vi "PlateReaderTimeTest.vi"() -> ()   [LabVIEW 2014]
uses:
  EventHandleInstrumentStatusChangedData.ctl
  EventHandleErrorReportData.ctl
  EventHandleCommandCompletedData.ctl
  C:/Program Files (x86)/Molecular Devices/SoftMax Pro 6.5.1 Automation SDK/SoftMaxPro.AutomationClient.dll
  Program Files (x86)/Molecular Devices/SoftMax Pro 6.5.1 Automation SDK/SoftMaxPro.AutomationClient.dll
  PlateReaderGlobal.vi
panel:
  out "Destruct Error":errorcluster
  out "String":string
  in  "ColumnName":string="1"
  out "Offsets":dbl[](array[numeric])
  in  "READ STOP":bool
  in  "READ START":bool
  in  "stop":bool
  out "Status":string
  out "ErrorReportQueue":T1[](array[typedef])
  out "CommandCompleteQueue":T2[](array[typedef])
  out "GetDataCopy":i32
  out "CommandCompleted":T2
  out "ErrorReport":T1
  out "InstrumentStatusChanged":T3
  out "StartRead":i32
  out "Initialize":bool
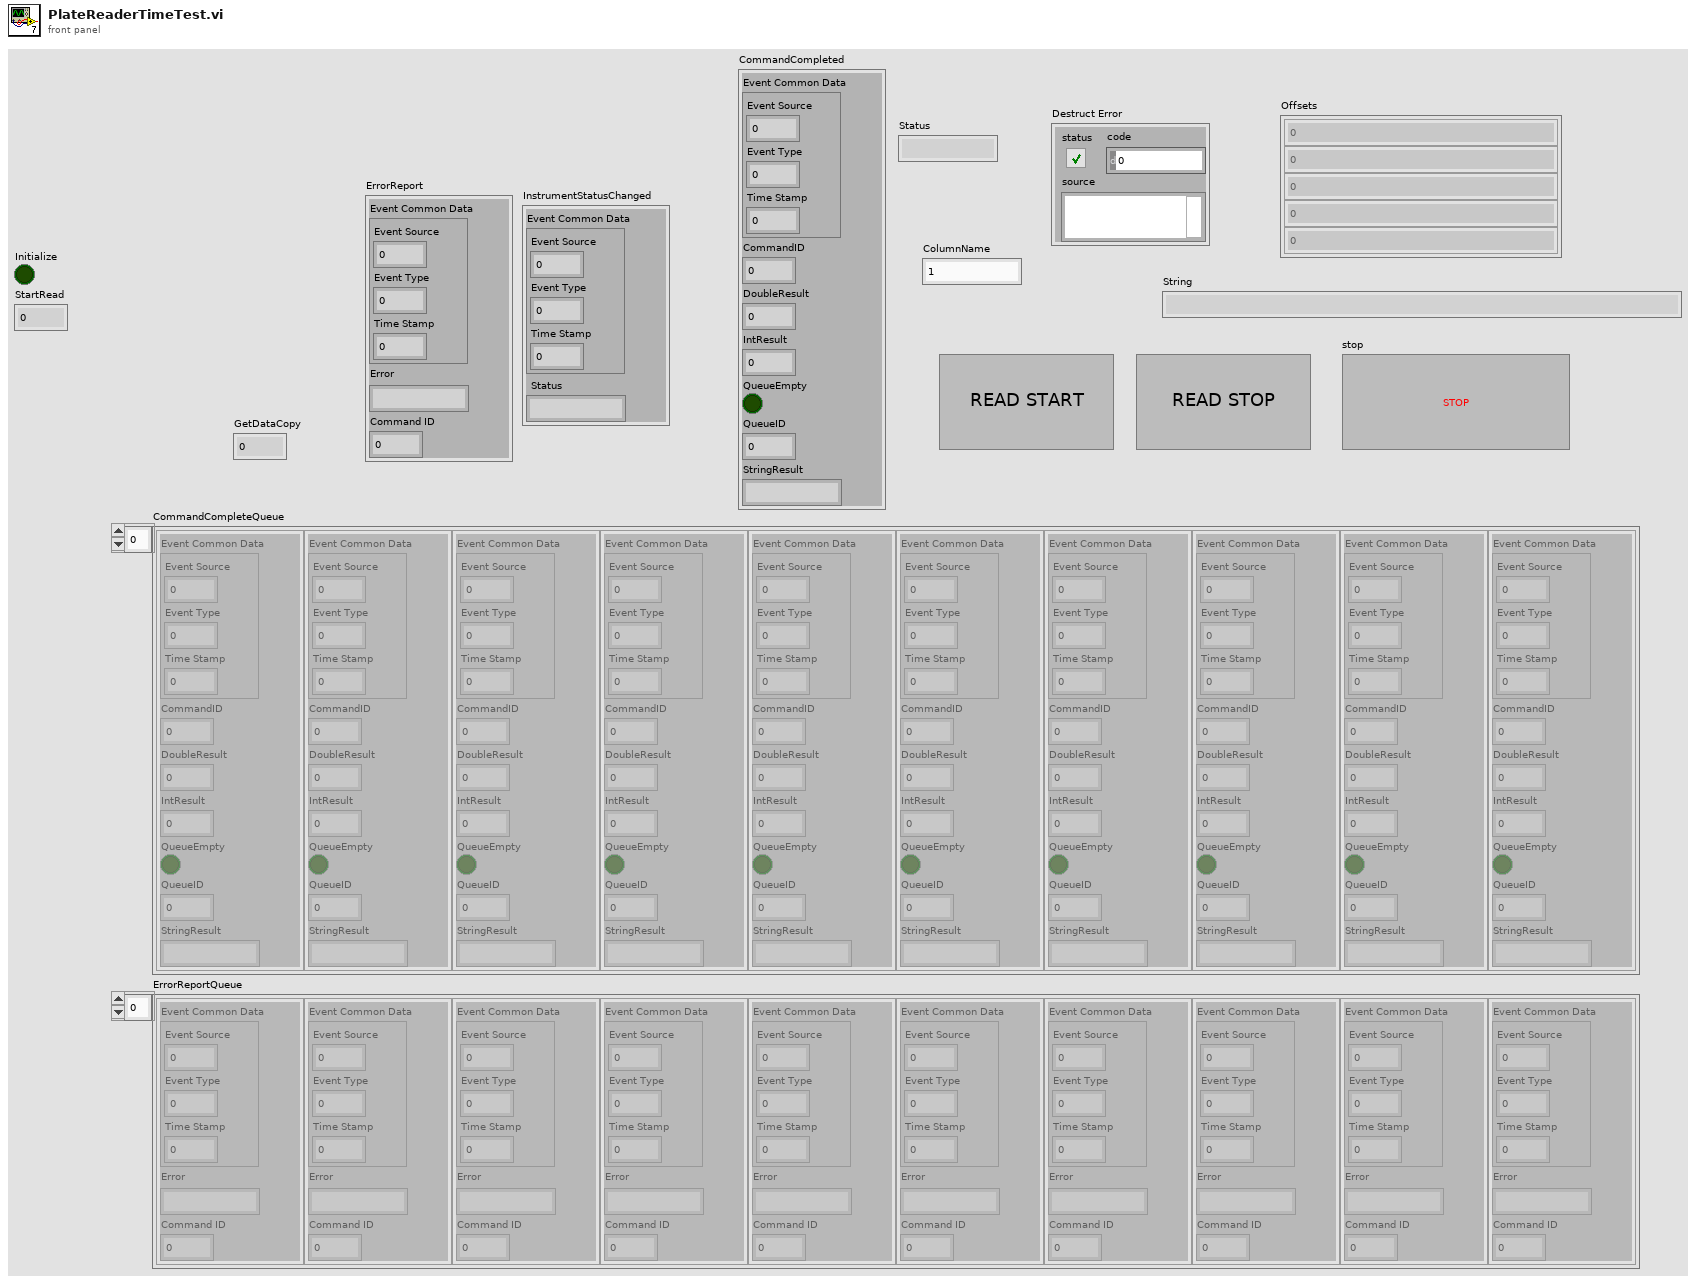
[diagram p1: front panel]
types:
  T1 = typedef "EventHandleErrorReportData.ctl" = cluster{"Event Common Data":cluster{"Event Source":i32, "Event Type":u32, "Time Stamp":u32}, "Error":string, "Command ID":i32}
  T2 = typedef "EventHandleCommandCompletedData.ctl" = cluster{"Event Common Data":cluster{"Event Source":i32, "Event Type":u32, "Time Stamp":u32}, "CommandID":i32, "DoubleResult":dbl, "IntResult":i32, "QueueEmpty":bool, "QueueID":i32, "StringResult":string}
  T3 = typedef "EventHandleInstrumentStatusChangedData.ctl" = cluster{"Event Common Data":cluster{"Event Source":i32, "Event Type":u32, "Time Stamp":u32}, "Status":string}
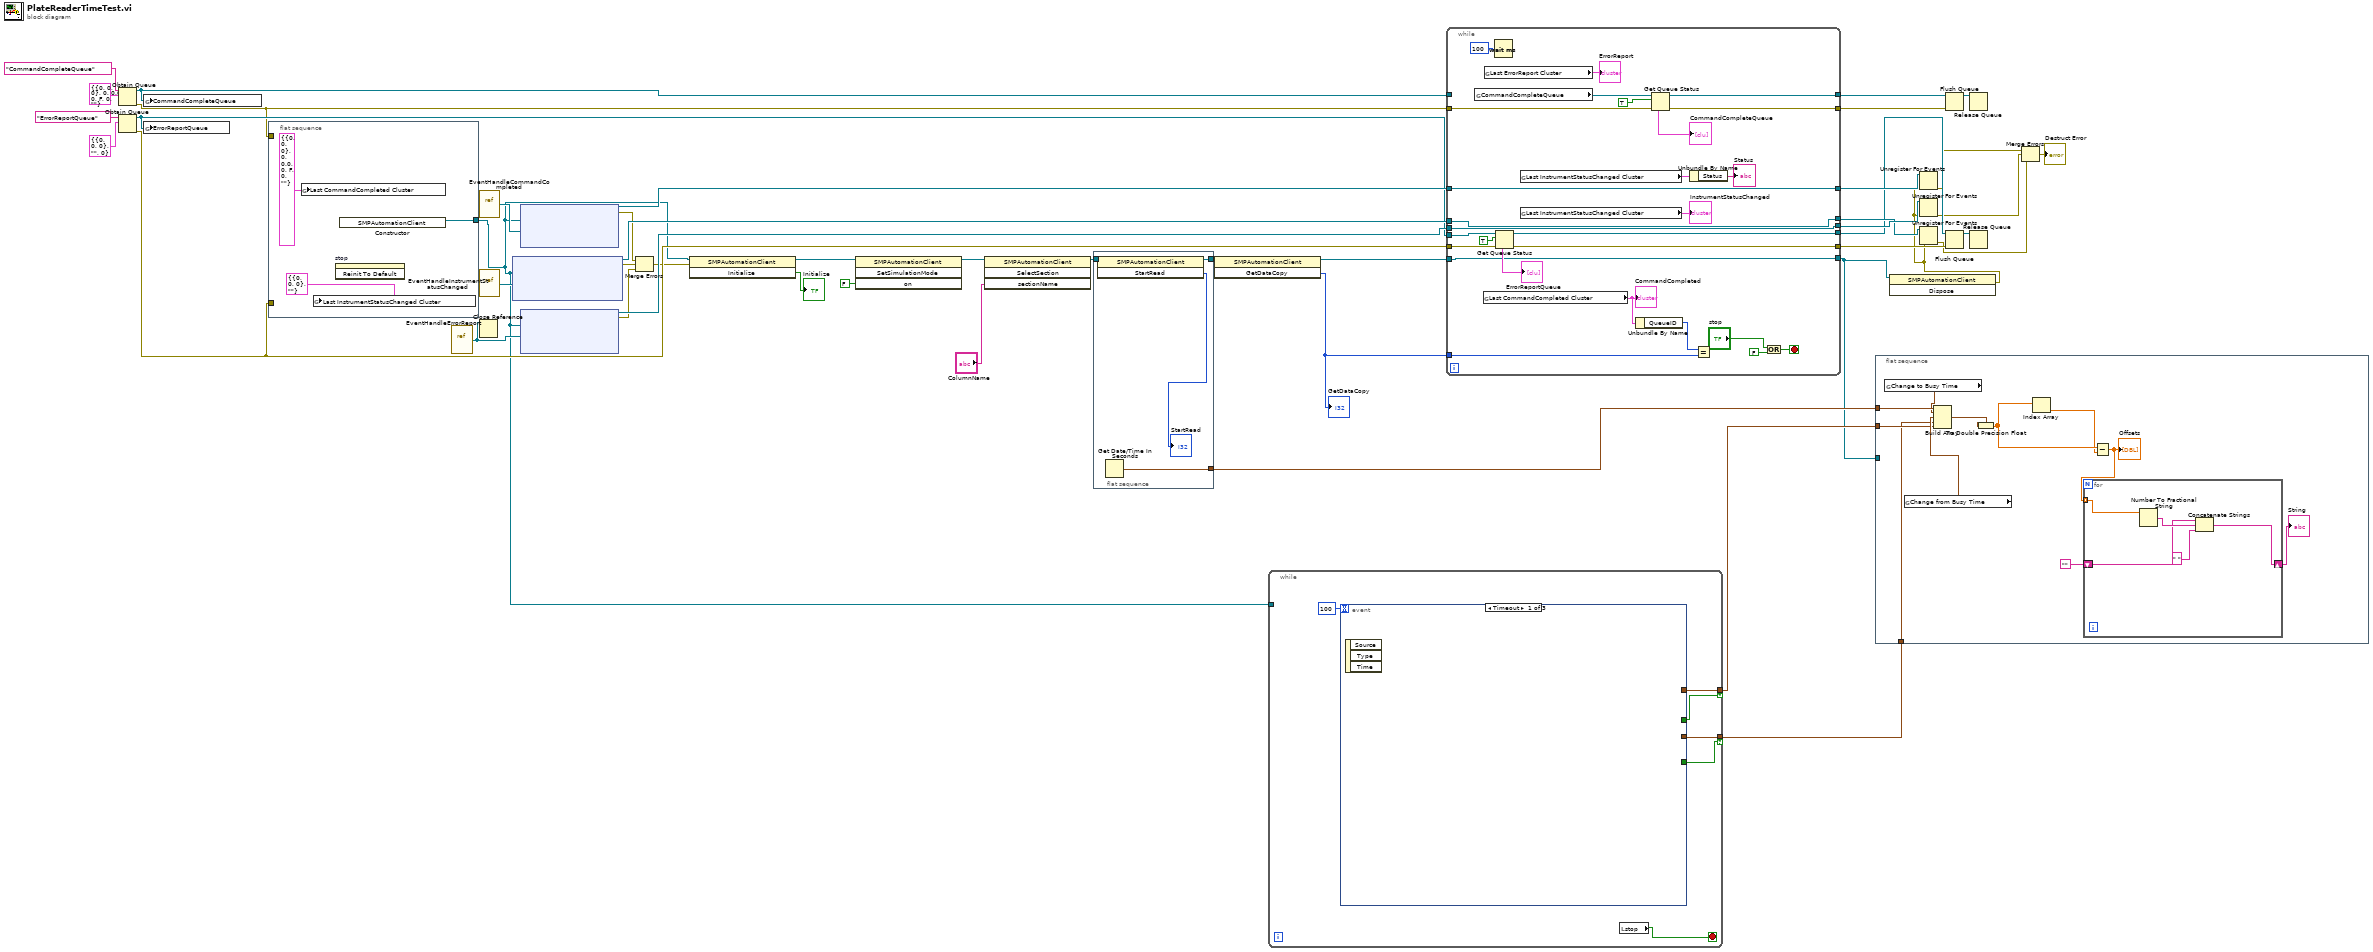
[diagram p0: block diagram]
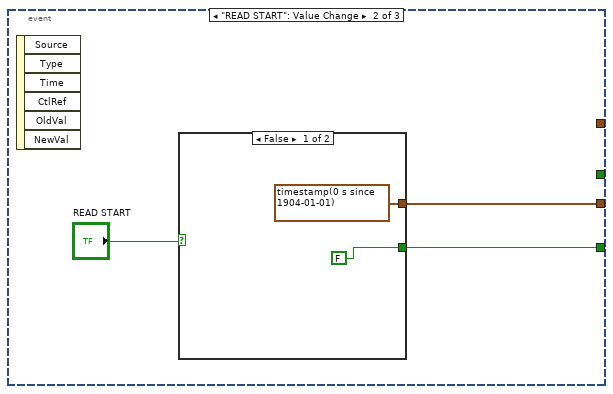
[diagram p2: hidden frame]
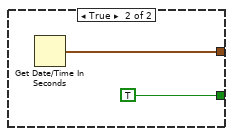
[diagram p3: hidden frame]
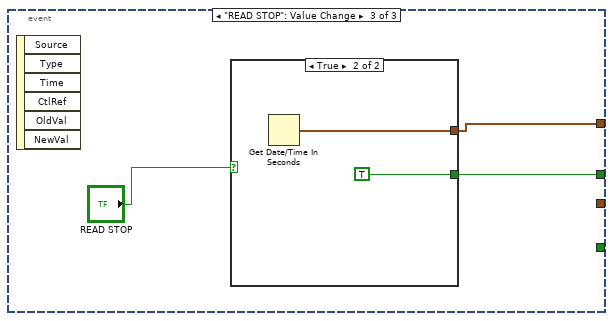
[diagram p4: hidden frame]
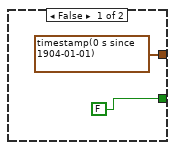
[diagram p5: hidden frame]
diagram:
  n1 = Obtain Queue(name (unnamed)="CommandCompleteQueue", element data type=T2 {"Event Common Data"={"Event Source"=0, "Event Type"=0, "Time Stamp"=0}, "CommandID"=0, "DoubleResult"=0.0, "IntResult"=0, "QueueEmpty"=FALSE, "QueueID"=0, "StringResult"=""} ("Event Data Cluster")) -> (queue out=w26:refnum<queue>, error out=w21:errorcluster)  [unwired: 3 in, 1 out]
  n2 = Obtain Queue(name (unnamed)="ErrorReportQueue", element data type=T1 {"Event Common Data"={"Event Source"=0, "Event Type"=0, "Time Stamp"=0}, "Error"="", "Command ID"=0} ("ErrorReport Data")) -> (queue out=w24:refnum<queue>, error out=w22:errorcluster)  [unwired: 3 in, 1 out]
  n3 = global write "PlateReaderGlobal.vi" "CommandCompleteQueue"(w26) -> ()
  n4 = global write "PlateReaderGlobal.vi" "ErrorReportQueue"(w24) -> ()
  n5 = flat-sequence {
    tunnel: [w49] -> w8
    tunnel: w22 -> [_]
    tunnel: w21 -> [_]
    frame #0 {
      n6 = global write "PlateReaderGlobal.vi" "Last CommandCompleted Cluster"(T2 {"Event Common Data"={"Event Source"=0, "Event Type"=0, "Time Stamp"=0}, "CommandID"=0, "DoubleResult"=0.0, "IntResult"=0, "QueueEmpty"=FALSE, "QueueID"=0, "StringResult"=""} ("Last CommandCompleted Cluster")) -> ()
      n7 = global write "PlateReaderGlobal.vi" "Last InstrumentStatusChanged Cluster"(T3 {"Event Common Data"={"Event Source"=0, "Event Type"=0, "Time Stamp"=0}, "Status"=""} ("Last InstrumentStatusChanged Cluster")) -> ()
      n8 = invoke on="stop" class="Bool (strict)" method="Reinit To Default"() -> ()  [unwired: 3 in, 3 out]
      n9 = constructor class="SMPAutomationClient"() -> (reference out=w49:refnum<k24>)  [unwired: 3 in, 2 out]
    }
  }
  n10 = vi-ref "EventHandleErrorReport.vi"() -> ("vi reference"=w35:refnum<vi>)
  n11 = vi-ref "EventHandleCommandCompleted.vi"() -> ("vi reference"=w40:refnum<vi>)
  n12 = vi-ref "EventHandleInstrumentStatusChanged.vi"() -> ("vi reference"=w39:refnum<vi>)
  n13 = Close Reference(reference=w35) -> ()  [unwired: 1 in, 1 out]
  n14 = node(w8, w39) -> (w41:refnum<k27>, w37:errorcluster)  [unwired: 3 in]
  n15 = node(w8, w40) -> (w45:refnum<k27>, w38:errorcluster)  [unwired: 3 in]
  n16 = node(w8, w35) -> (w43:refnum<k27>, w36:errorcluster)  [unwired: 3 in]
  n17 = Merge Errors(w38, w37, w36) -> (w20:errorcluster)
  n18 = invoke class="SMPAutomationClient" method="Initialize"(reference=w8, error in=w20) -> (reference out=w13:refnum<k24>, "Initialize"=→"Initialize":bool)  [unwired: 1 in, 1 out]
  n19 = invoke class="SMPAutomationClient" method="SetSimulationMode"(reference=w13, "on"=FALSE) -> (reference out=w17:refnum<k24>)  [unwired: 2 in, 3 out]
  n20 = invoke class="SMPAutomationClient" method="SelectSection"(reference=w17, "sectionName"="ColumnName") -> (reference out=w16:refnum<k24>)  [unwired: 2 in, 3 out]
  n21 = flat-sequence {
    tunnel: w16 -> [w53]
    tunnel: [w52] -> w15
    tunnel: [w50] -> w12
    frame #0 {
      n22 = invoke class="SMPAutomationClient" method="StartRead"(reference=w53) -> (reference out=w52:refnum<k24>, "StartRead"=→"StartRead":i32)  [unwired: 2 in, 1 out]
      n23 = Get Date/Time In Seconds() -> (seconds since 1Jan1904=w50:timestamp)
    }
  }
  n24 = invoke class="SMPAutomationClient" method="GetDataCopy"(reference=w15) -> (reference out=w7:refnum<k24>, "GetDataCopy"=w14:i32)  [unwired: 2 in, 1 out]
  "GetDataCopy" <- w14
  n25 = while {
    tunnel: [w60] -> w10 if=w59
    tunnel: [w58] -> w11 if=w57
    tunnel: [w54] -> _
    tunnel: w8 -> [w54]
    stop <- w56 stop-if-true
    n26 = event shown="[0] Timeout" {
      selector: _ -> [_ _ _]
      dyn-events: _ -> [_ _ _]
      timeout: 100 -> [_ _ _]
      tunnel: [_ w62 _] -> w60
      tunnel: [_ w61 _] -> w59
      tunnel: [_ _ w69] -> w58
      tunnel: [_ _ w68] -> w57
      event Timeout {
        n27 = event-data() -> ()  [unwired: 1 in, 3 out]
      }
      event "READ START": Value Change {
        n28 = event-data() -> ()  [unwired: 1 in, 6 out]
        n29 = case shown="False" "READ START" {
          tunnel: [timestamp(0 s since 1904-01-01) ("seconds since 1Jan1904") w67] -> w62
          tunnel: [FALSE TRUE] -> w61
          frame False {
          }
          frame True {
            n30 = Get Date/Time In Seconds() -> (seconds since 1Jan1904=w67:timestamp)
          }
        }
      }
      event "READ STOP": Value Change {
        n31 = event-data() -> ()  [unwired: 1 in, 6 out]
        n32 = case shown="True" "READ STOP" {
          tunnel: [timestamp(0 s since 1904-01-01) ("seconds since 1Jan1904") w74] -> w69
          tunnel: [FALSE TRUE] -> w68
          frame False {
          }
          frame True {
            n33 = Get Date/Time In Seconds() -> (seconds since 1Jan1904=w74:timestamp)
          }
        }
      }
    }
    n34 = local read "stop"() -> (w56:bool)
  }
  n35 = while {
    tunnel: [w101] -> w46
    tunnel: w45 -> [w101]
    tunnel: w7 -> [w76]
    tunnel: [w100] -> w44
    tunnel: w43 -> [w100]
    tunnel: [w99] -> w42
    tunnel: w41 -> [w99]
    tunnel: w21 -> [w92]
    tunnel: [w91] -> w28
    tunnel: w22 -> [w90]
    tunnel: [w89] -> w27
    tunnel: w26 -> [_]
    tunnel: [w88] -> w25
    tunnel: w24 -> [w87]
    tunnel: [w86] -> w23
    tunnel: w14 -> [w80]
    tunnel: [w76] -> w6
    stop <- w78 stop-if-true
    n36 = global read "PlateReaderGlobal.vi" "CommandCompleteQueue"() -> (w84:refnum<queue>)
    n37 = global read "PlateReaderGlobal.vi" "Last CommandCompleted Cluster"() -> (w81:T2)
    "CommandCompleted" <- w81
    n38 = global read "PlateReaderGlobal.vi" "Last ErrorReport Cluster"() -> (→"ErrorReport":T1)
    n39 = Wait (ms)(milliseconds to wait=u32 100) -> ()  [unwired: 1 out]
    n40 = Get Queue Status(queue=w87, return elements? (F)=TRUE, error in (no error)=w90) -> (queue out=w86:refnum<queue>, error out=w89:errorcluster, elements=→"ErrorReportQueue":T1[])  [unwired: 5 out]
    n41 = global read "PlateReaderGlobal.vi" "Last InstrumentStatusChanged Cluster"() -> (w93:T3)
    n42 = global read "PlateReaderGlobal.vi" "Last InstrumentStatusChanged Cluster"() -> (→"InstrumentStatusChanged":T3)
    n43 = Unbundle By Name(w81) -> ("QueueID"=w79:i32)
    n44 = Get Queue Status(queue=w84, return elements? (F)=TRUE, error in (no error)=w92) -> (queue out=w88:refnum<queue>, error out=w91:errorcluster, elements=→"CommandCompleteQueue":T2[])  [unwired: 5 out]
    n45 = Unbundle By Name(w93) -> ("Status"=→"Status":string)
    n46 = Equal?(x=w79, y=w80) -> ()  [unwired: 1 out]
    n47 = Or(x="stop", y=FALSE) -> (x .or. y?=w78:bool)
  }
  n48 = flat-sequence {
    tunnel: w6 -> [_]
    tunnel: w12 -> [w112]
    tunnel: w11 -> [w109]
    tunnel: w10 -> [w108]
    frame #0 {
      n49 = global read "PlateReaderGlobal.vi" "Change to Busy Time"() -> (w111:timestamp)
      n50 = global read "PlateReaderGlobal.vi" "Change from Busy Time"() -> (w110:timestamp)
      n51 = Build Array(w112, w111, w110, w108, w109) -> (w107:timestamp[])
      n52 = To Double Precision Float(number=w107) -> (double precision float=w106:dbl[])
      n53 = Index Array(array=w106) -> (element=w105:dbl)  [unwired: 1 in]
      n54 = Subtract(x=w106, y=w105) -> (x-y=w104:dbl[])
      "Offsets" <- w104
      n55 = for {
        tunnel: w104 -> [w117] mode=indexing
        shift-right: [w113] -> w102
        shift-left: "" -> [w114]
        n56 = Number To Fractional String(number=w117) -> (F-format string=w115:string)  [unwired: 3 in]
        n57 = Concatenate Strings(w114, w115, " " ("string")) -> (w113:string)
      }
      "String" <- w102
    }
  }
  n58 = invoke class="SMPAutomationClient" method="Dispose"(reference=w6) -> (error out=w5:errorcluster)  [unwired: 2 in, 2 out]
  n59 = Unregister For Events(event registration refnum=w46, error in=w5) -> (error out=w4:errorcluster)
  n60 = Unregister For Events(event registration refnum=w44, error in=w5) -> (error out=w3:errorcluster)
  n61 = Unregister For Events(event registration refnum=w42, error in=w5) -> (error out=w2:errorcluster)
  n62 = Flush Queue(queue=w25, error in (no error)=w28) -> (queue out=w30:refnum<queue>)  [unwired: 2 out]
  n63 = Flush Queue(queue=w23, error in (no error)=w27) -> (queue out=w29:refnum<queue>)  [unwired: 2 out]
  n64 = Release Queue(queue=w30) -> ()  [unwired: 2 in, 3 out]
  n65 = Release Queue(queue=w29) -> ()  [unwired: 2 in, 3 out]
  n66 = Merge Errors(w4, w3, w2) -> (→"Destruct Error":errorcluster)
